vi "write_ini.vi"(1 "Current OCT settings":T1) -> (0 "OCT settings out":T1)   [LabVIEW 2017]
doc: "Illustrates how to create and write a configuration settings file. Enter values in the controls on the front panel then click on the Run Arrow. To read the file, run Read Configuration (INI) File.vi."
uses:
  classes/HardwareObjects/Spectrometer/Spectrometer.lvclass
  classes/HardwareObjects/Camera/Camera.lvclass
  classes/HardwareObjects/DAQ/DAQ.lvclass
  classes/HardwareObjects/Galvonometer/Galvonometer.lvclass
  classes/HardwareObjects/PC/PC.lvclass
  classes/SoftwareObjects/ConfigProc/ConfigProc.lvclass
  classes/HardwareObjects/Spectrometer/Spectrometer.lvclass/Spectrometer.ctl
  classes/HardwareObjects/Camera/Camera.lvclass/Camera.ctl
  classes/HardwareObjects/DAQ/DAQ.lvclass/DAQ.ctl
  classes/HardwareObjects/Galvonometer/Galvonometer.lvclass/Galvonometer.ctl
  classes/HardwareObjects/PC/PC.lvclass/PC.ctl
  classes/SoftwareObjects/ConfigProc/ConfigProc.lvclass/ConfigProc.ctl
  classes/SoftwareObjects/ConfigProc/Read Blur Coefficient.vi
  classes/SoftwareObjects/ConfigProc/Read Blur Int.vi
  classes/SoftwareObjects/ConfigProc/Read Cores.vi
  classes/SoftwareObjects/ConfigProc/Read Interpolation.vi
  classes/SoftwareObjects/ConfigProc/Read Magnification.vi
  classes/SoftwareObjects/ConfigProc/Read Power.vi
  classes/SoftwareObjects/ConfigProc/Read Soften.vi
  classes/SoftwareObjects/ConfigProc/Read Weight.vi
  classes/HardwareObjects/PC/Read Max Number of Cores.vi
  classes/HardwareObjects/PC/Read Path to DLL.vi
  classes/HardwareObjects/Galvonometer/Read Make Model.vi
  classes/HardwareObjects/Galvonometer/Read Max Scan Angle (degrees).vi
  classes/HardwareObjects/Galvonometer/Read Output Scale Factor (V_degrees).vi
  classes/HardwareObjects/DAQ/Read Camera Counter.vi
  classes/HardwareObjects/DAQ/Read Camera Counter Output Terminal.vi
  classes/HardwareObjects/DAQ/Read Galvo Analog Output Channel(s).vi
  classes/HardwareObjects/DAQ/Read Galvo Counter.vi
  classes/HardwareObjects/DAQ/Read Galvo Counter Terminal.vi
  classes/HardwareObjects/DAQ/Read Master Counter.vi
  classes/HardwareObjects/DAQ/Read Master Counter Terminal.vi
  classes/HardwareObjects/Camera/Read Bit Depth.vi
  classes/HardwareObjects/Camera/Read Camera Dimensions.vi
  classes/HardwareObjects/Camera/Read Data Representation.vi
  classes/HardwareObjects/Camera/Read Duty Cycle.vi
  classes/HardwareObjects/Camera/Read Make, Model.vi
  classes/HardwareObjects/Camera/Read Max Frequency (kHz).vi
  classes/HardwareObjects/Camera/Read Return Time (us).vi
  classes/HardwareObjects/Spectrometer/Read Bandwidth (nm).vi
  classes/HardwareObjects/Spectrometer/Read Center wavelength (nm).vi
  classes/HardwareObjects/Spectrometer/Read Make Model.vi
  classes/HardwareObjects/Spectrometer/Read Scan depth (mm).vi
  <vilib>/Utility/config.llb/Write Key (String).vi
  <vilib>/Utility/config.llb/Write Key (Double).vi
  <vilib>/Utility/config.llb/NI_LVConfig.lvlib
panel:
  out "Processing Properties":T2
  out "PC Properties":T3
  out "Galvo Properties":T4
  out "DAQ Properties":T5
  out "Camera Properties":T6
  out "Label.Text":string
  out "Spectrometer Properties":T7
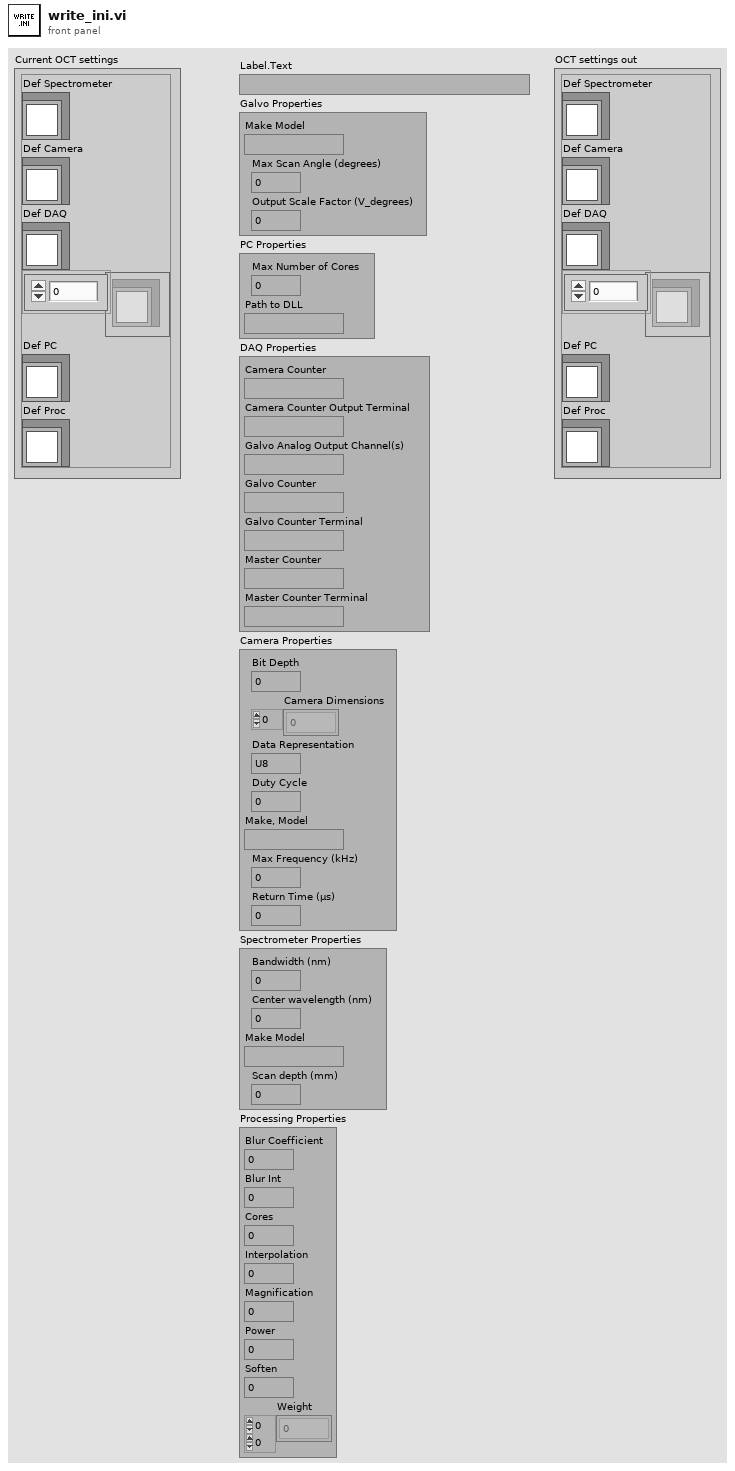
[diagram p1: front panel]
types:
  T1 = cluster{"Def Spectrometer":refnum<class "Spectrometer.lvclass">, "Def Camera":refnum<class "Camera.lvclass">, "Def DAQ":refnum<class "DAQ.lvclass">, "Array":refnum<class "Galvonometer.lvclass">[], "Def PC":refnum<class "PC.lvclass">, "Def Proc":refnum<class "ConfigProc.lvclass">}
  T2 = cluster{"Blur Coefficient":dbl, "Blur Int":dbl, "Cores":dbl, "Interpolation":dbl, "Magnification":dbl, "Power":dbl, "Soften":dbl, "Weight":cdb[][]}
  T3 = cluster{"Max Number of Cores":dbl, "Path to DLL":path}
  T4 = cluster{"Make Model":string, "Max Scan Angle (degrees)":dbl, "Output Scale Factor (V_degrees)":dbl}
  T5 = cluster{"Camera Counter":tag, "Camera Counter Output Terminal":tag, "Galvo Analog Output Channel(s)":tag, "Galvo Counter":tag, "Galvo Counter Terminal":tag, "Master Counter":tag, "Master Counter Terminal":tag}
  T6 = cluster{"Bit Depth":dbl, "Camera Dimensions":u16[], "Data Representation":enum16{"U8", "I8", "U16", "I16"}, "Duty Cycle":sgl, "Make, Model":string, "Max Frequency (kHz)":sgl, "Return Time (µs)":sgl}
  T7 = cluster{"Bandwidth (nm)":dbl, "Center wavelength (nm)":dbl, "Make Model":string, "Scan depth (mm)":dbl}
  T8 = typedef "NI_LVConfig.lvlib/Config Data RefNum.ctl" = refnum<k1>
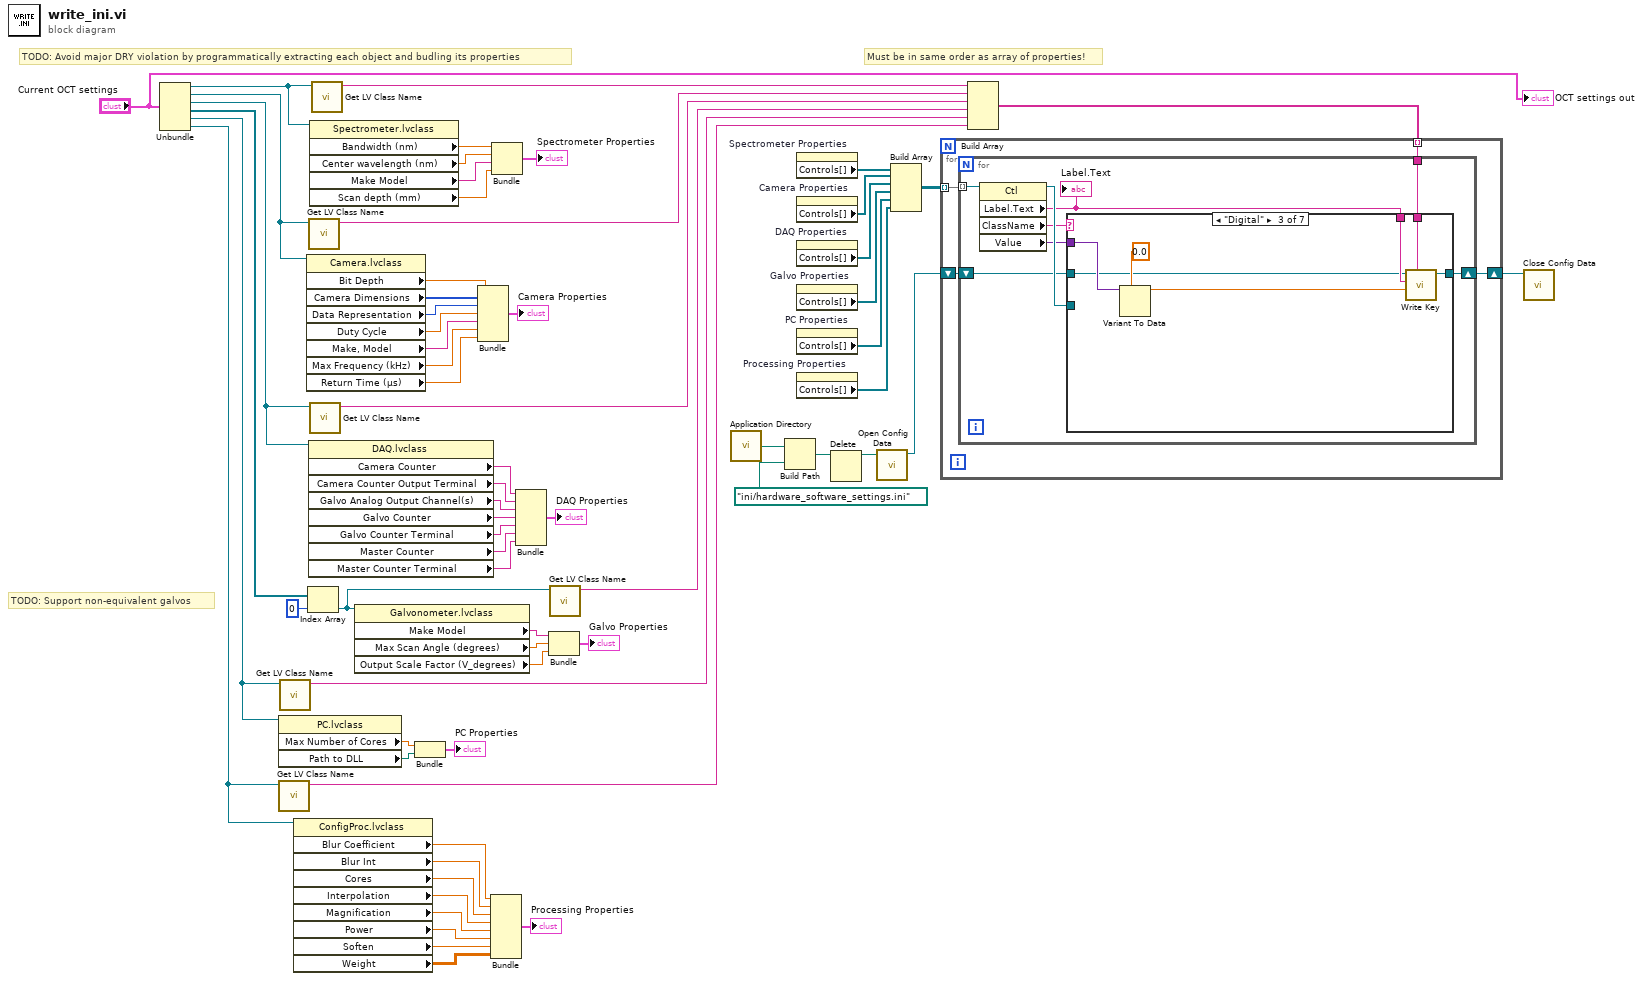
[diagram p0: block diagram]
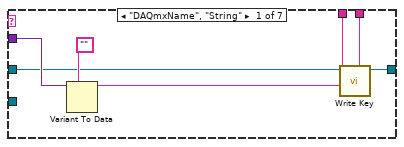
[diagram p2: hidden frame]
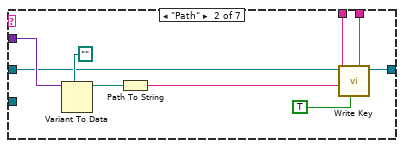
[diagram p3: hidden frame]
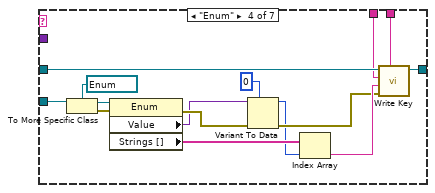
[diagram p4: hidden frame]
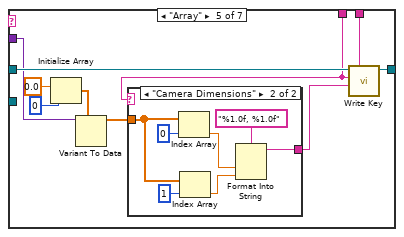
[diagram p5: hidden frame]
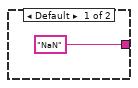
[diagram p6: hidden frame]
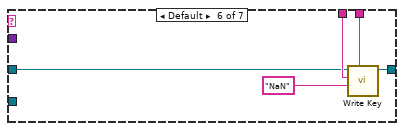
[diagram p7: hidden frame]
diagram:
  # "TODO: Support non-equivalent galvos"
  # "Must be in same order as array of properties!"
  # "TODO: Avoid major DRY violation by programmatically extracting each object and budling its properties"
  n1 = Unbundle("Current OCT settings") -> ("Def Spectrometer"=w66:refnum<class "Spectrometer.lvclass">, "Def Camera"=w48:refnum<class "Camera.lvclass">, "Def DAQ"=w39:refnum<class "DAQ.lvclass">, "Array"=w28:refnum<class "Galvonometer.lvclass">[], "Def PC"=w19:refnum<class "PC.lvclass">, "Def Proc"=w13:refnum<class "ConfigProc.lvclass">)
  n2 = property class="PC.lvclass"(reference=w19) -> ("Max Number of Cores"=w17:dbl, "Path to DLL"=w16:path)  [unwired: 1 in, 2 out]
  n3 = call <vilib>:"Get LV Class Name.vi"("object"=w13) -> ("class name"=w12:string)  [unwired: 9 in, 1 out]
  n4 = call <vilib>:"Get LV Class Name.vi"("object"=w19) -> ("class name"=w18:string)  [unwired: 9 in, 1 out]
  n5 = property class="ConfigProc.lvclass"(reference=w13) -> ("Blur Coefficient"=w11:dbl, "Blur Int"=w10:dbl, "Cores"=w9:dbl, "Interpolation"=w8:dbl, "Magnification"=w7:dbl, "Power"=w6:dbl, "Soften"=w5:dbl, "Weight"=w4:cdb[][])  [unwired: 1 in, 2 out]
  n6 = property class="Camera.lvclass"(reference=w48) -> ("Bit Depth"=w55:dbl, "Camera Dimensions"=w54:u16[], "Data Representation"=w53:enum16{"U8", "I8", "U16", "I16"}, "Duty Cycle"=w52:sgl, "Make, Model"=w51:string, "Max Frequency (kHz)"=w50:sgl, "Return Time (µs)"=w49:sgl)  [unwired: 1 in, 2 out]
  n7 = Index Array(array=w28, index=0) -> (element=w21:refnum<class "Galvonometer.lvclass">)
  n8 = call <vilib>:"Get LV Class Name.vi"("object"=w48) -> ("class name"=w42:string)  [unwired: 9 in, 1 out]
  n9 = property class="DAQ.lvclass"(reference=w39) -> ("Camera Counter"=w38:tag, "Camera Counter Output Terminal"=w37:tag, "Galvo Analog Output Channel(s)"=w36:tag, "Galvo Counter"=w35:tag, "Galvo Counter Terminal"=w34:tag, "Master Counter"=w33:tag, "Master Counter Terminal"=w32:tag)  [unwired: 1 in, 2 out]
  n10 = property class="Spectrometer.lvclass"(reference=w66) -> ("Bandwidth (nm)"=w65:dbl, "Center wavelength (nm)"=w64:dbl, "Make Model"=w63:string, "Scan depth (mm)"=w62:dbl)  [unwired: 1 in, 2 out]
  n11 = call <vilib>:"Get LV Class Name.vi"("object"=w39) -> ("class name"=w29:string)  [unwired: 9 in, 1 out]
  n12 = call <vilib>:"Get LV Class Name.vi"("object"=w66) -> ("class name"=w43:string)  [unwired: 9 in, 1 out]
  n13 = property class="Galvonometer.lvclass"(reference=w21) -> ("Make Model"=w26:string, "Max Scan Angle (degrees)"=w25:dbl, "Output Scale Factor (V_degrees)"=w24:dbl)  [unwired: 1 in, 2 out]
  n14 = Bundle("Max Number of Cores"=w17, "Path to DLL"=w16) -> (→"PC Properties":T3)  [unwired: 1 in]
  n15 = Bundle("Bit Depth"=w55, "Camera Dimensions"=w54, "Data Representation"=w53, "Duty Cycle"=w52, "Make, Model"=w51, "Max Frequency (kHz)"=w50, "Return Time (µs)"=w49) -> (→"Camera Properties":T6)  [unwired: 1 in]
  n16 = Bundle("Blur Coefficient"=w11, "Blur Int"=w10, "Cores"=w9, "Interpolation"=w8, "Magnification"=w7, "Power"=w6, "Soften"=w5, "Weight"=w4) -> (→"Processing Properties":T2)  [unwired: 1 in]
  n17 = Bundle("Bandwidth (nm)"=w65, "Center wavelength (nm)"=w64, "Make Model"=w63, "Scan depth (mm)"=w62) -> (→"Spectrometer Properties":T7)  [unwired: 1 in]
  n18 = Bundle("Camera Counter"=w38, "Camera Counter Output Terminal"=w37, "Galvo Analog Output Channel(s)"=w36, "Galvo Counter"=w35, "Galvo Counter Terminal"=w34, "Master Counter"=w33, "Master Counter Terminal"=w32) -> (→"DAQ Properties":T5)  [unwired: 1 in]
  n19 = Bundle("Make Model"=w26, "Max Scan Angle (degrees)"=w25, "Output Scale Factor (V_degrees)"=w24) -> (→"Galvo Properties":T4)  [unwired: 1 in]
  n20 = call <vilib>:"Get LV Class Name.vi"("object"=w21) -> ("class name"=w20:string)  [unwired: 9 in, 1 out]
  n21 = call <vilib>:"Application Directory.vi"() -> ("Application Directory"=w57:path)
  n22 = Build Path(base path=w57, name or relative path=path "ini/hardware_software_settings.ini" ("default name")) -> (appended path=w58:path)
  n23 = property on="Spectrometer Properties" class="Clust (strict)"() -> ("Controls[]"=w46:refnum<vi>[])  [unwired: 2 in, 2 out]
  n24 = property on="Camera Properties" class="Clust (strict)"() -> ("Controls[]"=w45:refnum<vi>[])  [unwired: 2 in, 2 out]
  n25 = property on="DAQ Properties" class="Clust (strict)"() -> ("Controls[]"=w30:refnum<vi>[])  [unwired: 2 in, 2 out]
  n26 = property on="Galvo Properties" class="Clust (strict)"() -> ("Controls[]"=w22:refnum<vi>[])  [unwired: 2 in, 2 out]
  n27 = property on="PC Properties" class="Clust (strict)"() -> ("Controls[]"=w14:refnum<vi>[])  [unwired: 2 in, 2 out]
  n28 = property on="Processing Properties" class="Clust (strict)"() -> ("Controls[]"=w2:refnum<vi>[])  [unwired: 2 in, 2 out]
  n29 = Delete(path (use dialog)=w58) -> (deleted path=w59:path)  [unwired: 4 in, 2 out]
  n30 = call <vilib>:"Open Config Data.vi"("configuration file path"=w59) -> ("refnum"=w56:T8)  [unwired: 2 in, 8 out]
  n31 = Build Array(w46, w45, w30, w22, w14, w2) -> (w44:refnum<vi>[][])
  n32 = Build Array(w43, w42, w29, w20, w18, w12) -> (w41:string[])
  n33 = for {
    tunnel: w41 -> [w70] mode=indexing
    tunnel: w44 -> [w68] mode=indexing
    shift-right: [w67] -> w40
    shift-left: w56 -> [w69]
    n34 = for {
      tunnel: w68 -> [w77] mode=indexing
      tunnel: w70 -> [w72]
      shift-right: [w71] -> w67
      shift-left: w69 -> [w73]
      n35 = property class="Ctl"(reference=w77) -> (reference out=w78:refnum<vi>, "Label.Text"=w74:string, "ClassName"=w76:string, "Value"=w75:variant)  [unwired: 1 in, 1 out]
      "Label.Text" <- w74
      n36 = case shown="\"Digital\"" w76 {
        tunnel: w75 -> [w85 w93 w101 _ w123 _ _]
        tunnel: w72 -> [w83 w89 w96 w114 w126 w135 _]
        tunnel: w74 -> [w82 w90 w98 w113 w119 w138 _]
        tunnel: w73 -> [w80 w92 w97 w116 w125 w137 w140]
        tunnel: [w79 w91 w95 w115 w124 w136 w140] -> w71
        tunnel: w78 -> [_ _ _ w110 _ _ _]
        frame "DAQmxName", "String" {
          n37 = Variant To Data(type="", Variant=w85) -> (data=w81:string)  [unwired: 1 in, 1 out]
          n38 = call-poly <vilib>:"Write Key.vi"("section"=w83, "value"=w81, "key"=w82, "refnum"=w80) -> ("refnum out"=w79:T8)  [unwired: 5 in, 2 out]
        }
        frame "Path" {
          n39 = Variant To Data(type=path "", Variant=w93) -> (data=w88:path)  [unwired: 1 in, 1 out]
          n40 = Path To String(path=w88) -> (string=w87:string)
          n41 = call-poly <vilib>:"Write Key.vi"("write raw string? (F)"=TRUE, "section"=w89, "value"=w87, "key"=w90, "refnum"=w92) -> ("refnum out"=w91:T8)  [unwired: 4 in, 2 out]
        }
        frame "Digital" {
          n42 = Variant To Data(type=0.0, Variant=w101) -> (data=w99:dbl)  [unwired: 1 in, 1 out]
          n43 = call-poly <vilib>:"Write Key.vi"("section"=w96, "value"=w99, "key"=w98, "refnum"=w97) -> ("refnum out"=w95:T8)  [unwired: 5 in, 2 out]
        }
        frame "Enum" {
          n44 = To More Specific Class(target class=refnum<vi> refnum ("TESTITEM"), reference=w110) -> (specific class reference=w109:refnum<vi>, error out=w108:errorcluster)  [unwired: 1 in]
          n45 = property class="Enum"(reference=w109, error in=w108) -> (error out=w107:errorcluster, "Value"=w106:variant, "Strings []"=w105:string[])  [unwired: 1 out]
          n46 = Variant To Data(error in=w107, type=0, Variant=w106) -> (data=w102:i32, error out=w103:errorcluster)
          n47 = Index Array(array=w105, index=w102) -> (element=w104:string)
          n48 = call-poly <vilib>:"Write Key.vi"("section"=w114, "error in (no error)"=w103, "value"=w104, "key"=w113, "refnum"=w116) -> ("refnum out"=w115:T8)  [unwired: 4 in, 2 out]
        }
        frame "Array" {
          n49 = Initialize Array(0.0 ("element"), 0 ("dimension size")) -> (w120:dbl[])
          n50 = Variant To Data(type=w120, Variant=w123) -> (data=w117:dbl[])  [unwired: 1 in, 1 out]
          n51 = case shown="\"Camera Dimensions\"" w119 {
            tunnel: ["NaN" w128] -> w118
            tunnel: w117 -> [_ w133]
            frame Default {
            }
            frame "Camera Dimensions" {
              n52 = Index Array(array=w133, index=0) -> (element=w130:dbl)
              n53 = Index Array(array=w133, index=1) -> (element=w129:dbl)
              n54 = Format Into String(format string="%1.0f, %1.0f", w130, w129) -> (resulting string=w128:string)  [unwired: 2 in, 1 out]
            }
          }
          n55 = call-poly <vilib>:"Write Key.vi"("section"=w126, "value"=w118, "key"=w119, "refnum"=w125) -> ("refnum out"=w124:T8)  [unwired: 5 in, 2 out]
        }
        frame Default {
          n56 = call-poly <vilib>:"Write Key.vi"("section"=w135, "value"="NaN", "key"=w138, "refnum"=w137) -> ("refnum out"=w136:T8)  [unwired: 5 in, 2 out]
        }
        frame "" {
        }
      }
    }
  }
  n57 = call <vilib>:"Close Config Data.vi"("refnum"=w40) -> ()  [unwired: 2 in, 9 out]
  "OCT settings out" <- "Current OCT settings"
